vi "打开程序.vi"(8 "error in (no error)":errorcluster caption="错误输入（无错误）", 11 "程序 输入":refnum<class "程序.lvclass">) -> (0 "error out":errorcluster caption="错误输出", 3 "程序 输出":refnum<class "程序.lvclass">)   [LabVIEW 2018, in "程序.lvclass"]
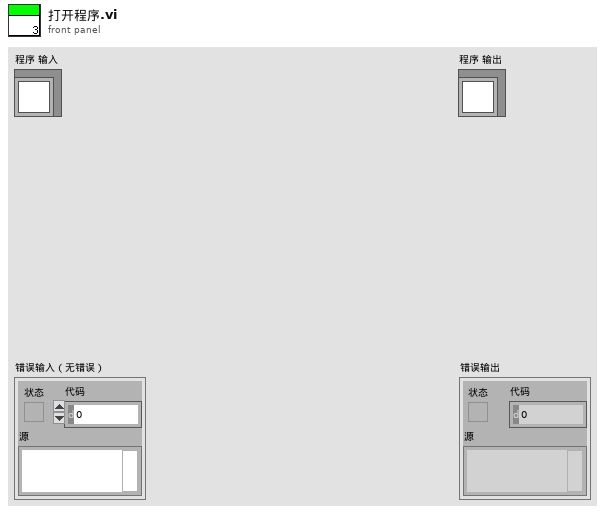
[diagram p1: front panel]
types:
  T1 = typedef "imagedata.ctl" = cluster{"image type":i32, "image depth":i32, "image":u8[], "mask":u8[], "colors":u32[], "Rectangle":cluster{"left":i16, "top":i16, "right":i16, "bottom":i16}}
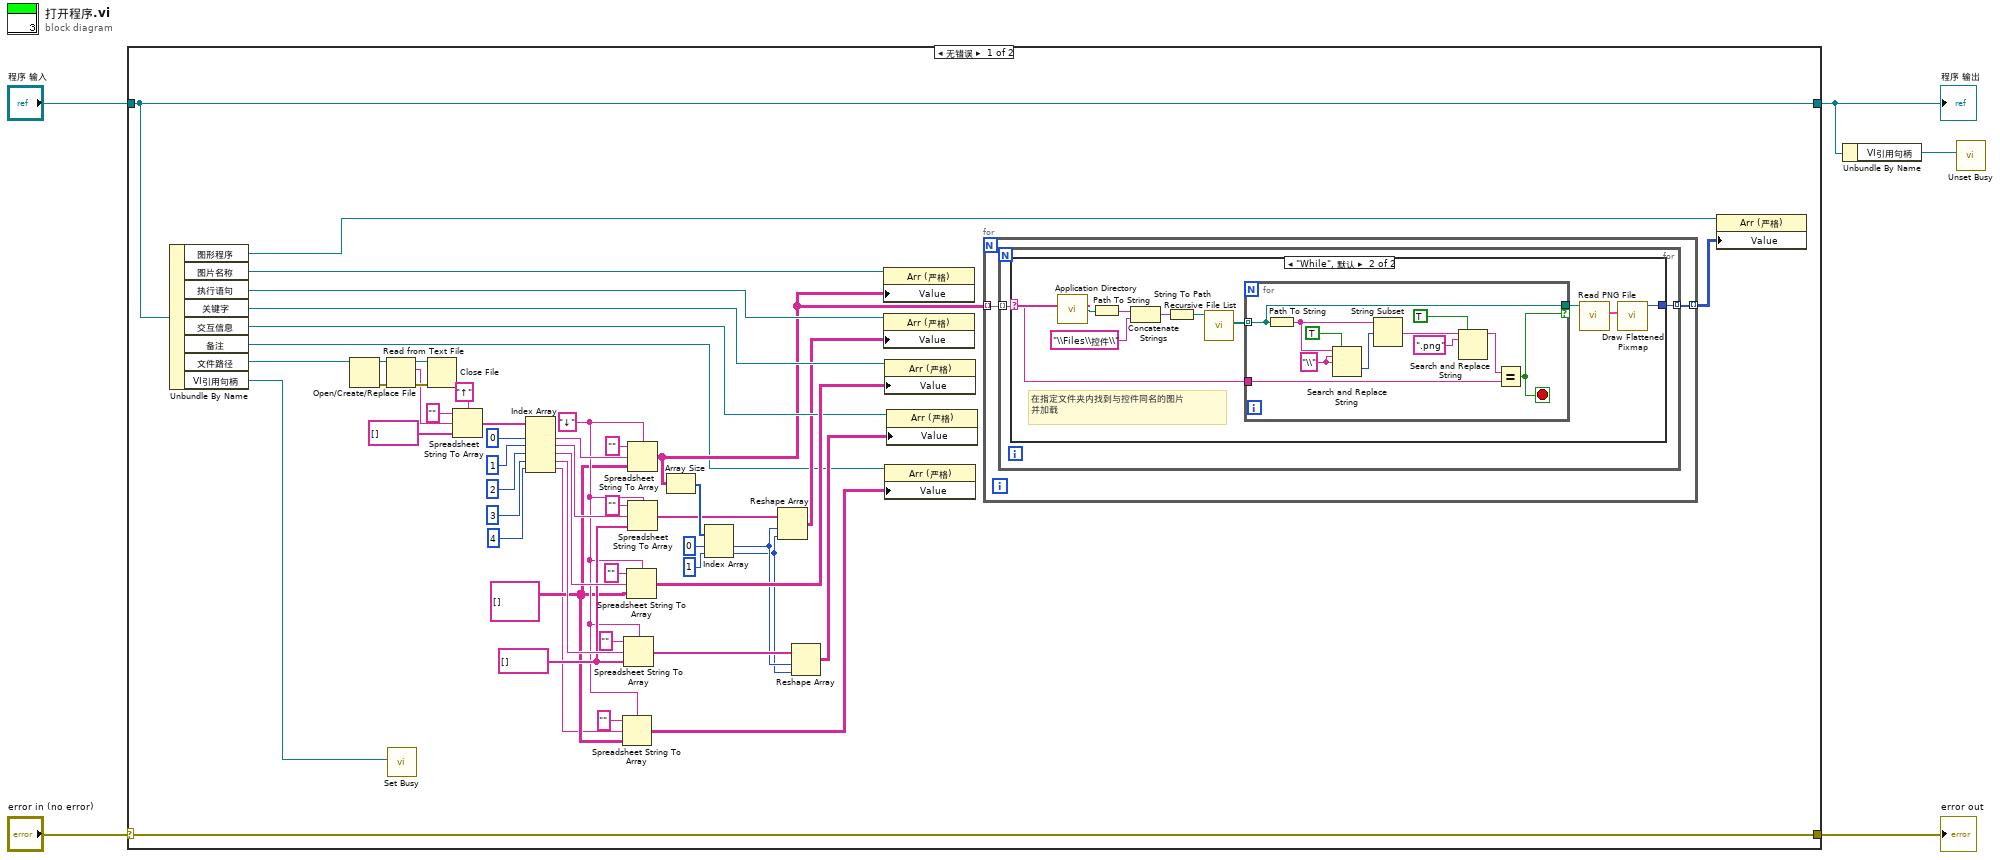
[diagram p0: block diagram]
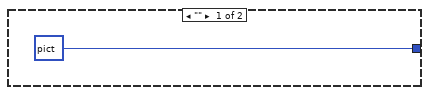
[diagram p2: hidden frame]
diagram:
  n1 = case shown="无错误" "error in (no error)" {
    selector: "error in (no error)" -> [w55 w83]
    tunnel: [w55 w83] -> w4
    tunnel: [w50 w82] -> w2
    tunnel: "程序 输入" -> [w50 w82]
    frame No Error {
      w11 = "↓" ("分隔符(Tab)")
      w19 = string[] []
      w10 = string[][] []
      n2 = Unbundle By Name(w50) -> ("图形程序"=w31:refnum<vi>, "图片名称"=w40:refnum<vi>, "执行语句"=w33:refnum<vi>, "关键字"=w32:refnum<vi>, "交互信息"=w25:refnum<vi>, "备注"=w8:refnum<vi>, "文件路径"=w49:path, "VI引用句柄"=w6:refnum<vi>)
      n3 = Open/Create/Replace File(file path (use dialog)=w49) -> (refnum out=w54:refnum<file>, error out=w53:errorcluster)  [unwired: 5 in, 1 out]
      n4 = Read from Text File(file (use dialog)=w54, error in=w53) -> (refnum out=w52:refnum<file>, text=w45:string, error out=w51:errorcluster)  [unwired: 2 in, 1 out]
      n5 = call <vilib>:"Set Busy.vi"("VI reference (current VI)"=w6) -> ()  [unwired: 9 in, 2 out]
      n6 = Close File(refnum=w52, error in=w51) -> ()  [unwired: 2 out]
      n7 = Spreadsheet String To Array(delimiter (Tab)="↑" ("分隔符(Tab)"), format string="" ("格式字符串"), spreadsheet string=w45, array type (2D Dbl)=string[] []) -> (array=w44:string[])
      n8 = Index Array(array=w44, index #1=0 ("索引"), index #2=1 ("索引"), index #3=2 ("索引"), index #4=3 ("索引"), index #5=4 ("索引")) -> (element #1=w38:string, element #2=w37:string, element #3=w34:string, element #4=w26:string, element #5=w9:string)
      n9 = Spreadsheet String To Array(delimiter (Tab)=w11, format string="" ("格式字符串"), spreadsheet string=w9, array type (2D Dbl)=w10) -> (array=w7:string[][])
      n10 = Spreadsheet String To Array(delimiter (Tab)=w11, format string="" ("格式字符串"), spreadsheet string=w26, array type (2D Dbl)=w19) -> (array=w23:string[])
      n11 = Spreadsheet String To Array(delimiter (Tab)=w11, format string="" ("格式字符串"), spreadsheet string=w34, array type (2D Dbl)=w10) -> (array=w30:string[][])
      n12 = Spreadsheet String To Array(delimiter (Tab)=w11, format string="" ("格式字符串"), spreadsheet string=w38, array type (2D Dbl)=w10) -> (array=w24:string[][])
      n13 = Spreadsheet String To Array(delimiter (Tab)=w11, format string="" ("格式字符串"), spreadsheet string=w37, array type (2D Dbl)=w19) -> (array=w17:string[])
      n14 = Array Size(array=w24) -> (size(s)=w22:i32[])
      n15 = Index Array(array=w22, index #1=0 ("索引"), index #2=1 ("索引")) -> (element #1=w15:i32, element #2=w14:i32)
      n16 = Reshape Array(w17, w15, w14) -> (w16:string[][])
      n17 = Reshape Array(w23, w15, w14) -> (w18:string[][])
      n18 = property class="Arr (严格)"(reference=w40, "Value"=w24) -> ()  [unwired: 1 in, 2 out]
      n19 = property class="Arr (严格)"(reference=w33, "Value"=w16) -> ()  [unwired: 1 in, 2 out]
      n20 = property class="Arr (严格)"(reference=w32, "Value"=w30) -> ()  [unwired: 1 in, 2 out]
      n21 = property class="Arr (严格)"(reference=w8, "Value"=w7) -> ()  [unwired: 1 in, 2 out]
      n22 = property class="Arr (严格)"(reference=w25, "Value"=w18) -> ()  [unwired: 1 in, 2 out]
      n23 = for {
        tunnel: w24 -> [w57] mode=indexing
        tunnel: [w56] -> w29 mode=indexing
        n24 = for {
          tunnel: w57 -> [w59] mode=indexing
          tunnel: [w58] -> w56 mode=indexing
          n25 = case shown="\"While\", 默认" w59 {
            selector: w59 -> [_ w62]
            tunnel: [picture data[5B] ("二维图片") w69] -> w58
            frame "" {
            }
            frame "While", Default {
              # "在指定文件夹内找到与控件同名的图片\n并加载"
              n26 = call <vilib>:"Application Directory.vi"() -> ("Application Directory"=w63:path)
              n27 = Path To String(path=w63) -> (string=w66:string)
              n28 = Concatenate Strings(w66, "\\Files\\控件\\" ("名称或相对路径")) -> (w65:string)
              n29 = String To Path(string=w65) -> (path=w67:path)
              n30 = call <vilib>:"Recursive File List.vi"("Folder Path"=w67) -> ("All Files in Dir"=w68:path[])  [unwired: 6 in, 4 out]
              n31 = for {
                tunnel: w68 -> [w74] mode=indexing
                tunnel: [w74] -> w61 if=w71
                tunnel: w62 -> [w72]
                stop <- w71 stop-if-true
                w80 = "\\" ("搜索字符串")
                n32 = Path To String(path=w74) -> (string=w79:string)
                n33 = Search and Replace String(replace all?=TRUE ("替换全部？(F)"), input string=w79, search string=w80, replace string=w80) -> (offset past replacement=w78:i32)  [unwired: 4 in, 3 out]
                n34 = String Subset(string=w79, offset (0)=w78) -> (substring=w76:string)  [unwired: 1 in]
                n35 = Search and Replace String(replace all?=TRUE ("替换全部？(F)"), input string=w76, search string=".png" ("搜索字符串")) -> (result string=w73:string)  [unwired: 5 in, 3 out]
                n36 = Equal?(x=w73, y=w72) -> (x = y?=w71:bool)
              }
              n37 = call <vilib>:"Read PNG File.vi"("path to PNG file"=w61) -> ("image data"=w70:T1)  [unwired: 8 in, 2 out]
              n38 = call <vilib>:"Draw Flattened Pixmap.vi"("image data"=w70) -> ("new picture"=w69:picture)  [unwired: 8 in]
            }
          }
        }
      }
      n39 = property class="Arr (严格)"(reference=w31, "Value"=w29) -> ()  [unwired: 1 in, 2 out]
    }
    frame Error {
    }
  }
  "error out" <- w4
  "程序 输出" <- w2
  n40 = Unbundle By Name(w2) -> ("VI引用句柄"=w1:refnum<vi>)
  n41 = call <vilib>:"Unset Busy.vi"("VI reference (current VI)"=w1) -> ()  [unwired: 10 in, 1 out]
